vi "TestSkill.vi"(8 "error in (no error)":errorcluster, 10 "Robot":refnum<class "Robot.lvclass">, 11 "Skill in":refnum<class "TestSkill.lvclass">) -> (0 "error out":errorcluster, 2 "Robot out":refnum<class "Robot.lvclass">, 3 "Skill out":refnum<class "TestSkill.lvclass">)   [LabVIEW 2020, in "TestSkill.lvclass"]
uses:
  TestSkill.lvclass
  Robot_class/Robot.lvclass
  Robot_class/Robot.lvclass/Robot.ctl
  Robot_class/Write dest_x.vi
  Robot_class/Write dest_y.vi
  Robot_class/Write dest_orientation.vi
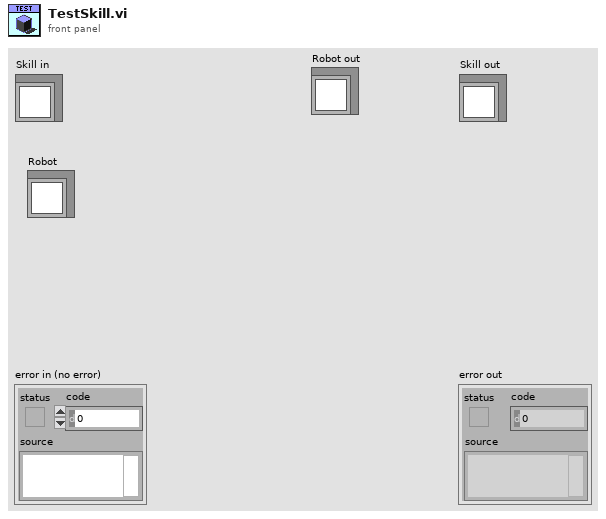
[diagram p1: front panel]
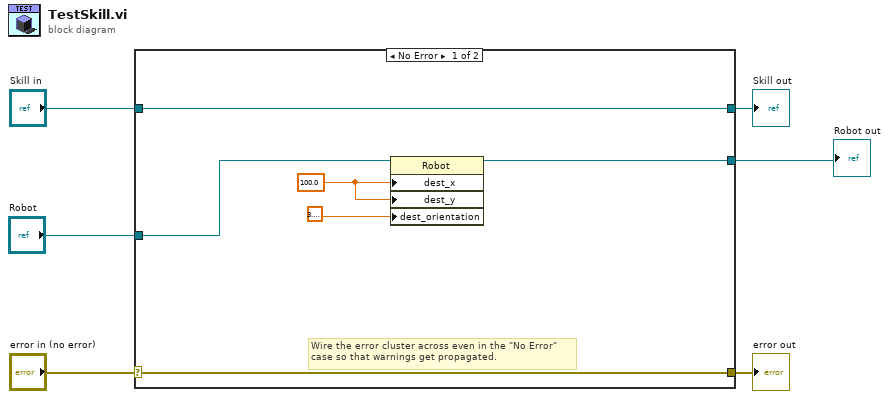
[diagram p0: block diagram]
diagram:
  n1 = case shown="No Error" "error in (no error)" {
    selector: "error in (no error)" -> [w11 w15]
    tunnel: [w11 w15] -> w5
    tunnel: [w12 w14] -> w3
    tunnel: "Skill in" -> [w12 w14]
    tunnel: "Robot" -> [w10 w13]
    tunnel: [w9 w13] -> w1
    frame No Error {
      w8 = 100.0 ("dest_x")
      # "Wire the error cluster across even in the \"No Error\"\ncase so that warnings get propagated."
      n2 = property class="Robot"(reference=w10, "dest_x"=w8, "dest_y"=w8, "dest_orientation"=3.141592653589793) -> (reference out=w9:refnum<class "Robot.lvclass">)  [unwired: 1 in, 1 out]
    }
    frame Error {
    }
  }
  "error out" <- w5
  "Skill out" <- w3
  "Robot out" <- w1
